vi "Drive Train Logger.vi"   [LabVIEW 2013]
uses:
  Drive Train Metrics.ctl
  CmdFlag.ctl
types:
  T1 = enum16{"open", "replace", "create", "open or create", "replace or create", "replace or create with confirmation"}
  T2 = typedef "Drive Train Metrics.ctl" = cluster{"last time in gear":u32, "Shift":bool, "Right Joystick":dbl, "Left Joystick":dbl, "CmdFlag":T3, "Right Motor Power":dbl, "Left Motor Power":dbl, "Right Accel.":dbl, "Left Accel.":dbl, "Filtered Left Drive Rate":dbl, "Filtered Right Drive Rate":dbl, "Direction of travel":enum16{"Backward", "Forward", "Spin"}, "AverageAccelleration":dbl, "Time of Last Metric":u32, "Time Of Last Shift":dbl, "Average Drive Rate":dbl, "Average Throttle":dbl, "FIFO Timeout":i32}
  T3 = typedef "CmdFlag.ctl" = enum16{"noop", "suspend", "resume"}
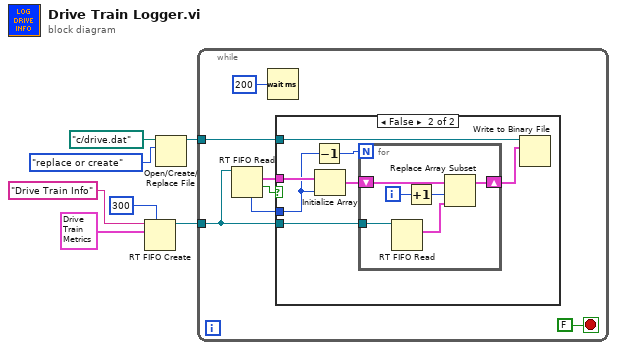
[diagram p0: block diagram]
diagram:
  n1 = RT FIFO Create(0:"Drive Train Info" ("name (unnamed)"), 1:T2 {"last time in gear"=0, "Shift"=FALSE, "Right Joystick"=0.0, "Left Joystick"=0.0, "CmdFlag"=enum."noop", "Right Motor Power"=0.0, "Left Motor Power"=0.0, "Right Accel."=0.0, "Left Accel."=0.0, "Filtered Left Drive Rate"=0.0, "Filtered Right Drive Rate"=0.0, "Direction of travel"=enum."Backward", "AverageAccelleration"=0.0, "Time of Last Metric"=0, "Time Of Last Shift"=0.0, "Average Drive Rate"=0.0, "Average Throttle"=0.0, "FIFO Timeout"=0} ("Cluster"), 4:300) -> (8:w2:refnum<k33>)  [unwired: 5 in, 2 out]
  n2 = Open/Create/Replace File(file path (use dialog)=path "c:/drive.dat", operation (0:open)=T1."replace or create") -> (refnum out=w7:refnum<file>)  [unwired: 4 in, 2 out]
  n3 = while {
    tunnel: w2 -> [w11]
    tunnel: w7 -> [w12]
    stop <- FALSE stop-if-true
    n4 = RT FIFO Read(0:w11) -> (7:w10:u32, 9:w9:T2, 10:w8:bool)  [unwired: 3 in, 2 out]
    n5 = Wait (ms)(milliseconds to wait=u32 200) -> ()  [unwired: 1 out]
    n6 = case shown="False" w8 {
      tunnel: w12 -> [_ w21]
      tunnel: w11 -> [_ w20]
      tunnel: w10 -> [_ w15]
      tunnel: w9 -> [_ w19]
      frame True {
      }
      frame False {
        n7 = Decrement(x=w15) -> (x-1=w16:u32)
        n8 = Initialize Array(w19, w15) -> (w18:T2[])
        n9 = for {
          N: w16 -> [_]
          tunnel: w20 -> [w27]
          shift-right: [w22] -> w17
          shift-left: w18 -> [w23]
          i -> [w25]
          n10 = RT FIFO Read(0:w27) -> (9:w26:T2)  [unwired: 3 in, 4 out]
          n11 = Increment(x=w25) -> (x+1=w24:i32)
          n12 = Replace Array Subset(array=w23, new element=w26, index=w24) -> (w22:T2[])
        }
        n13 = Write to Binary File(file (use dialog)=w21, data=w17) -> ()  [unwired: 4 in, 3 out]
      }
    }
  }
